vi "SVI increment ANODE array (SubVI).vi"(1 "End Voltage (V)":dbl, 2 "Increment Voltage (V)":dbl, 3 "Start Voltage (V)":dbl) -> (0 "output":dbl[](array[numeric]))   [LabVIEW 2020]
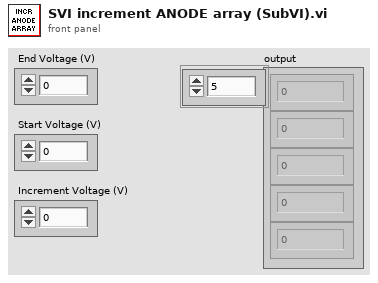
[diagram p1: front panel]
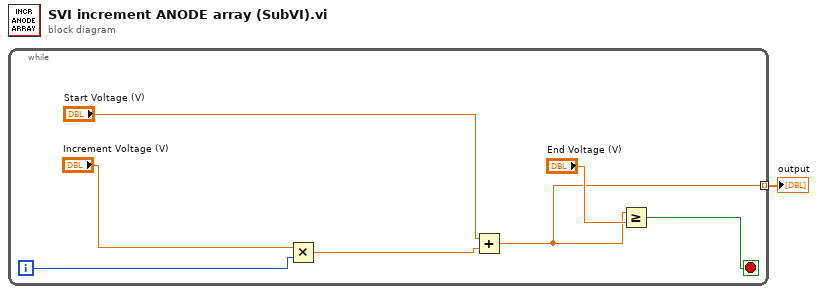
[diagram p0: block diagram]
diagram:
  n1 = while {
    tunnel: [w2] -> w1 mode=indexing
    i -> [w7]
    stop <- w3 stop-if-true
    n2 = Multiply(x="Increment Voltage (V)", y=w7) -> (x*y=w5:dbl)
    n3 = Add(x="Start Voltage (V)", y=w5) -> (x+y=w2:dbl)
    n4 = Greater Or Equal?(x=w2, y="End Voltage (V)") -> (x >= y?=w3:bool)
  }
  "output" <- w1
